vi "ENPH 354 Assignment 1 - Q1.vi"() -> ()   [LabVIEW 2021]
uses:
  <vilib>/numeric/Random Number (Range) U64.vi
  <vilib>/numeric/sub_Random U32.vi
panel:
  out "Average":dbl
  out "Array":dbl[](array[numeric])
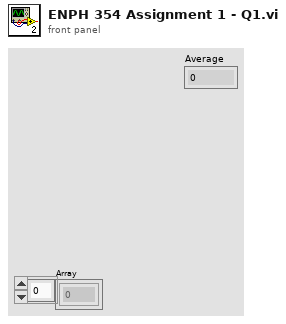
[diagram p1: front panel]
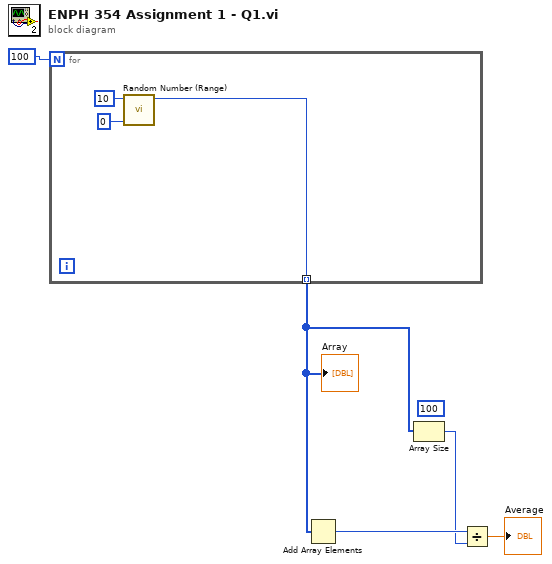
[diagram p0: block diagram]
diagram:
  (unwired) 100 ("size(s)")
  n1 = for {
    N: 100 -> [_]
    tunnel: [w6] -> w4 mode=indexing
    n2 = call-poly <vilib>:"Random Number (Range).vi"("lower bound (0)"=u64 0, "upper bound (100)"=u64 10) -> ("number"=w6:u64)  [unwired: 9 in]
  }
  "Array" <- w4
  n3 = Add Array Elements(numeric array=w4) -> (sum=w3:u64)
  n4 = Array Size(array=w4) -> (size(s)=w2:i32)
  n5 = Divide(x=w3, y=w2) -> (x/y=→"Average":dbl)
